vi "静态标定判定.vi"(7 "静态标定判定条件":T1={"主信号"={"单位"="", "下限"=49.6, "上限"=50.4}, "副信号"={"单位"="", "下限"=49.6, "上限"=50.4}, "主副和"={"单位"="", "下限"=99.2, "上限"=100.8}, "主副差"={"单位"="", "下限"=0.0, "上限"=0.8}, "Vres"={"单位"="", "下限"=96.0, "上限"=100.0}}, 9 "Vres":dbl, 10 "T2(%)":dbl, 11 "T1(%)":dbl) -> (3 "OK？":bool)   [LabVIEW 2020]
uses:
  Global_Variable/Global.vi
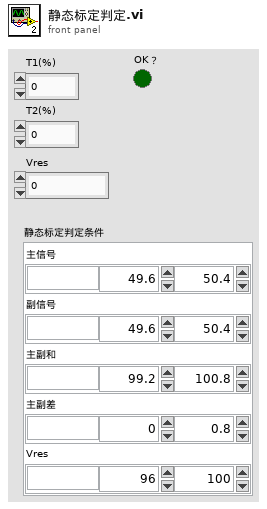
[diagram p1: front panel]
types:
  T1 = cluster{"主信号":cluster{"单位":string, "下限":dbl, "上限":dbl}, "副信号":cluster{"单位":string, "下限":dbl, "上限":dbl}, "主副和":cluster{"单位":string, "下限":dbl, "上限":dbl}, "主副差":cluster{"单位":string, "下限":dbl, "上限":dbl}, "Vres":cluster{"单位":string, "下限":dbl, "上限":dbl}}
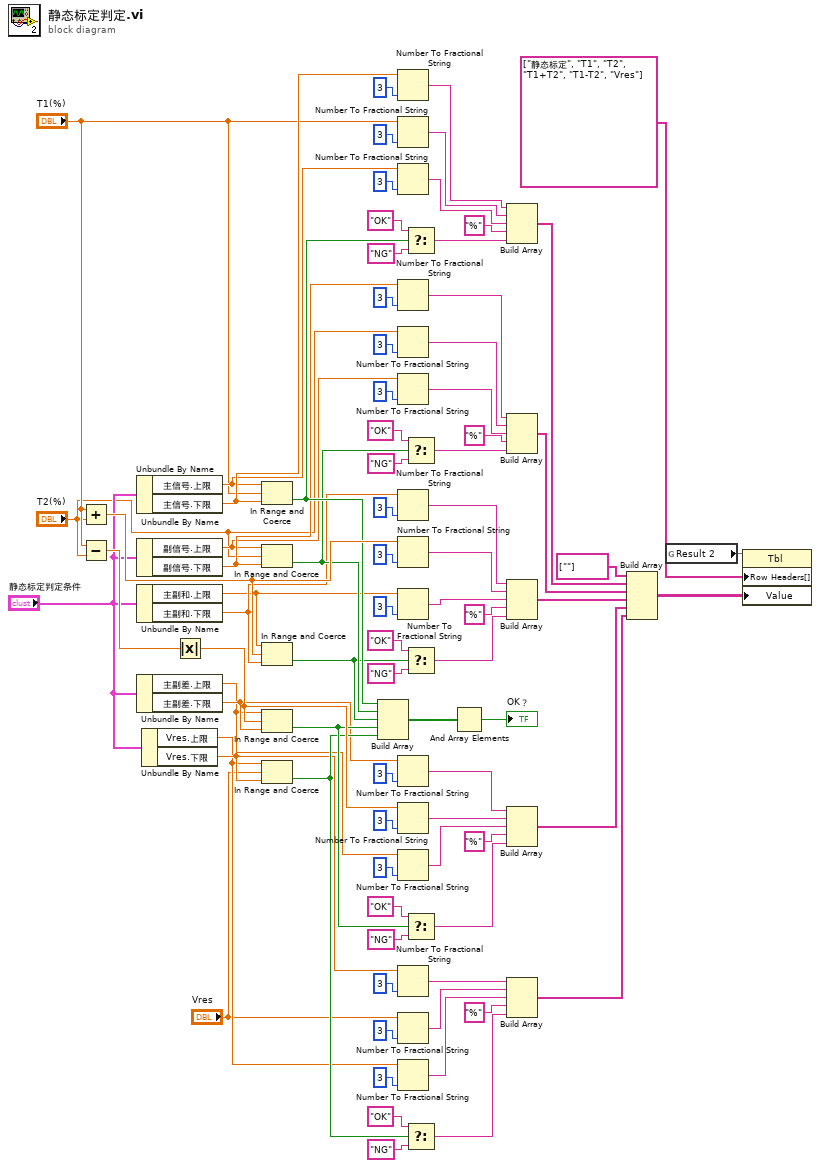
[diagram p0: block diagram]
diagram:
  n1 = Add(x="T1(%)", y="T2(%)") -> (x+y=w75:dbl)
  n2 = Subtract(x="T1(%)", y="T2(%)") -> (x-y=w40:dbl)
  n3 = Unbundle By Name("静态标定判定条件") -> ("主信号.上限"=w22:dbl, "主信号.下限"=w24:dbl)
  n4 = Unbundle By Name("静态标定判定条件") -> ("副信号.上限"=w19:dbl, "副信号.下限"=w20:dbl)
  n5 = Unbundle By Name("静态标定判定条件") -> ("主副和.上限"=w15:dbl, "主副和.下限"=w16:dbl)
  n6 = Unbundle By Name("静态标定判定条件") -> ("主副差.上限"=w13:dbl, "主副差.下限"=w14:dbl)
  n7 = Unbundle By Name("静态标定判定条件") -> ("Vres.上限"=w11:dbl, "Vres.下限"=w12:dbl)
  n8 = Absolute Value(x=w40) -> (abs(x)=w37:dbl)
  n9 = In Range and Coerce(upper limit=w22, x="T1(%)", lower limit=w24) -> (In Range?=w51:bool)  [unwired: 1 out]
  n10 = In Range and Coerce(upper limit=w19, x="T2(%)", lower limit=w20) -> (In Range?=w50:bool)  [unwired: 1 out]
  n11 = In Range and Coerce(upper limit=w15, x=w75, lower limit=w16) -> (In Range?=w49:bool)  [unwired: 1 out]
  n12 = In Range and Coerce(upper limit=w13, x=w37, lower limit=w14) -> (In Range?=w36:bool)  [unwired: 1 out]
  n13 = In Range and Coerce(upper limit=w11, x="Vres", lower limit=w12) -> (In Range?=w35:bool)  [unwired: 1 out]
  n14 = Build Array(w51, w50, w49, w36, w35) -> (w48:bool[])
  n15 = Number To Fractional String(number=w24, precision (6)=i16 3 ("精度(6)")) -> (F-format string=w23:string)  [unwired: 2 in]
  n16 = Number To Fractional String(number="T1(%)", precision (6)=i16 3 ("精度(6)")) -> (F-format string=w74:string)  [unwired: 2 in]
  n17 = Number To Fractional String(number=w22, precision (6)=i16 3 ("精度(6)")) -> (F-format string=w21:string)  [unwired: 2 in]
  n18 = Number To Fractional String(number=w20, precision (6)=i16 3 ("精度(6)")) -> (F-format string=w18:string)  [unwired: 2 in]
  n19 = Number To Fractional String(number="T2(%)", precision (6)=i16 3 ("精度(6)")) -> (F-format string=w68:string)  [unwired: 2 in]
  n20 = Number To Fractional String(number=w19, precision (6)=i16 3 ("精度(6)")) -> (F-format string=w17:string)  [unwired: 2 in]
  n21 = Number To Fractional String(number=w16, precision (6)=i16 3 ("精度(6)")) -> (F-format string=w10:string)  [unwired: 2 in]
  n22 = Number To Fractional String(number=w75, precision (6)=i16 3 ("精度(6)")) -> (F-format string=w62:string)  [unwired: 2 in]
  n23 = Number To Fractional String(number=w15, precision (6)=i16 3 ("精度(6)")) -> (F-format string=w9:string)  [unwired: 2 in]
  n24 = Number To Fractional String(number=w14, precision (6)=i16 3 ("精度(6)")) -> (F-format string=w8:string)  [unwired: 2 in]
  n25 = Number To Fractional String(number=w37, precision (6)=i16 3 ("精度(6)")) -> (F-format string=w45:string)  [unwired: 2 in]
  n26 = Number To Fractional String(number=w13, precision (6)=i16 3 ("精度(6)")) -> (F-format string=w7:string)  [unwired: 2 in]
  n27 = Number To Fractional String(number=w12, precision (6)=i16 3 ("精度(6)")) -> (F-format string=w6:string)  [unwired: 2 in]
  n28 = Number To Fractional String(number="Vres", precision (6)=i16 3 ("精度(6)")) -> (F-format string=w58:string)  [unwired: 2 in]
  n29 = Number To Fractional String(number=w11, precision (6)=i16 3 ("精度(6)")) -> (F-format string=w5:string)  [unwired: 2 in]
  n30 = Select(t="OK", s=w51, f="NG") -> (s? t:f=w72:string)
  n31 = Select(t="OK", s=w50, f="NG") -> (s? t:f=w71:string)
  n32 = Select(t="OK", s=w49, f="NG") -> (s? t:f=w63:string)
  n33 = Select(t="OK", s=w36, f="NG") -> (s? t:f=w44:string)
  n34 = Select(t="OK", s=w35, f="NG") -> (s? t:f=w61:string)
  n35 = And Array Elements(Boolean array=w48) -> (logical AND=→"OK？":bool)
  n36 = Build Array(w23, w74, w21, "%", w72) -> (w56:string[])
  n37 = Build Array(w18, w68, w17, "%", w71) -> (w55:string[])
  n38 = Build Array(w10, w62, w9, "%", w63) -> (w54:string[])
  n39 = Build Array(w8, w45, w7, "%", w44) -> (w38:string[])
  n40 = Build Array(w6, w58, w5, "%", w61) -> (w53:string[])
  n41 = Build Array(string[] [""] ("元素"), w56, w55, w54, w38, w53) -> (w52:string[][])
  n42 = global read "Global.vi" "Result 2"() -> (w83)
  n43 = property class="Tbl"(reference=w83, "Row Headers[]"=string[] ["静态标定", "T1", "T2", "T1+T2", "T1-T2", "Vres"] ("行首字符串[]"), "Value"=w52) -> ()  [unwired: 1 in, 2 out]
